vi "Continue Read.vi"(8 "error in":errorcluster, 11 "Com in":refnum<visa-resource-name>) -> (0 "error out":errorcluster, 2 "Data":i64[](array[numeric]), 3 "Com out":refnum<visa-resource-name>)   [LabVIEW 2020]
panel:
  out "read buffer":string
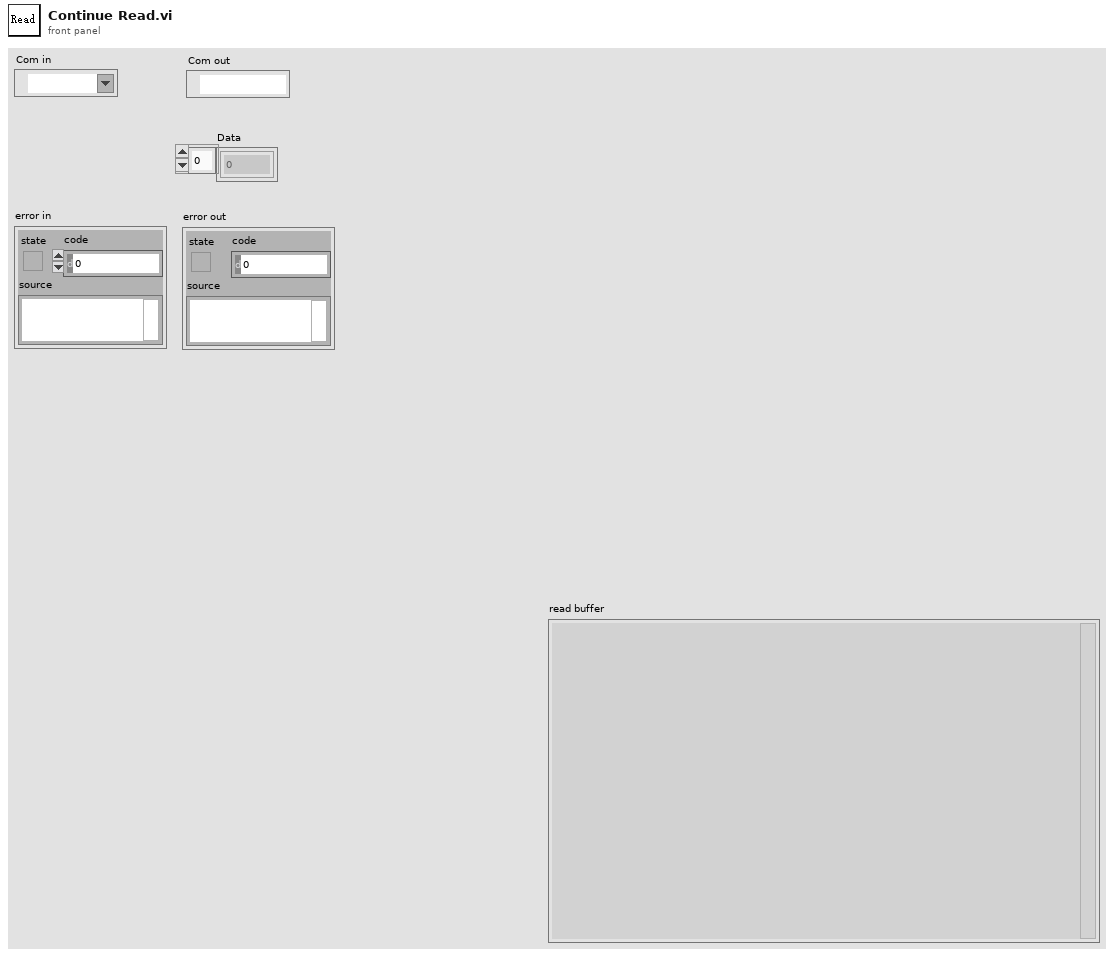
[diagram p1: front panel]
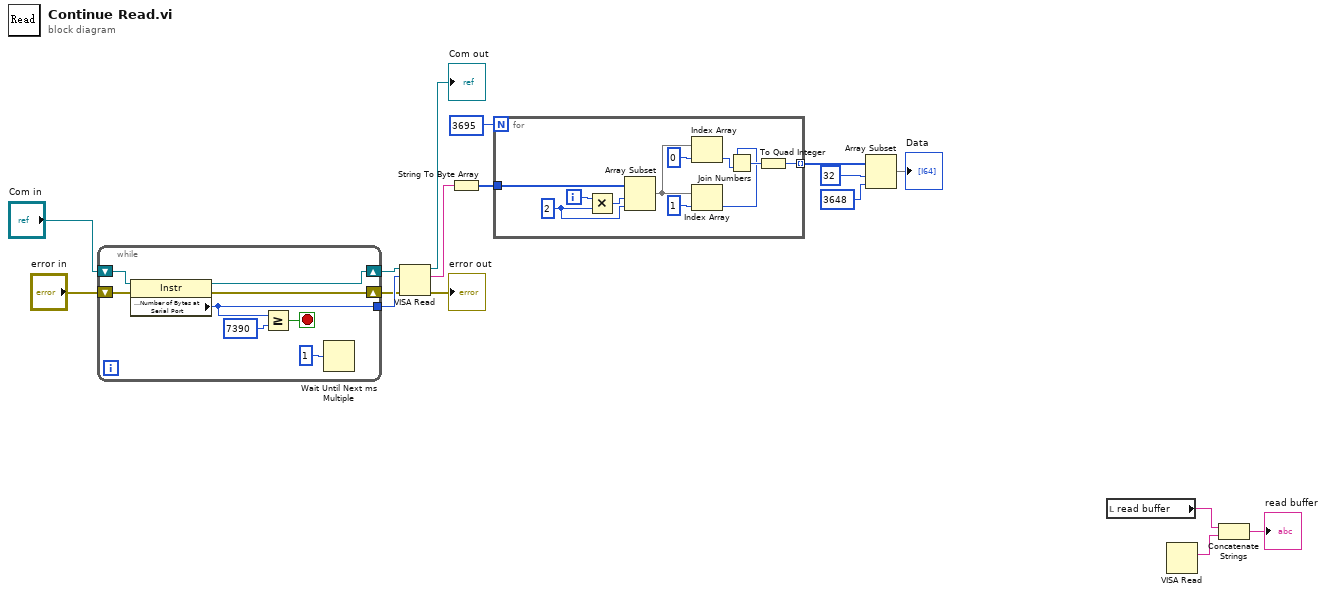
[diagram p0: block diagram]
diagram:
  n1 = while {
    tunnel: [w23] -> w18
    shift-right: [w26] -> w17
    shift-left: "error in" -> [w25]
    shift-right: [w27] -> w19
    shift-left: "Com in" -> [w24]
    stop <- w22 stop-if-true
    n2 = property class="Instr"(reference=w24, error in=w25) -> (reference out=w27:refnum<visa-resource-name>, error out=w26:errorcluster, "Serial Settings:Number of Bytes at Serial Port"=w23:u32)
    n3 = Greater Or Equal?(x=w23, y=u32 7390) -> (x >= y?=w22:bool)
    n4 = Wait Until Next ms Multiple(millisecond multiple=u32 1 ("毫秒倍数")) -> ()  [unwired: 1 out]
  }
  n5 = VISA Read(VISA resource name=w19, byte count=w18, error in (no error)=w17) -> (VISA resource name out=→"Com out":refnum<visa-resource-name>, read buffer=w16:string, error out=→"error out":errorcluster)  [unwired: 1 out]
  n6 = String To Byte Array(string=w16) -> (unsigned byte array=w15:u8[])
  n7 = for {
    N: 3695 -> [_]
    tunnel: w15 -> [w38]
    tunnel: [w30] -> w13 mode=indexing
    i -> [w36]
    w35 = 2 ("长度")
    n8 = Multiply(x=w36, y=w35) -> (x*y=w37:i32)
    n9 = Array Subset(array=w38, index=w37, length=w35) -> (w34:u8[])
    n10 = Index Array(array=w34, index=0 ("索引")) -> (element=w29:u8)
    n11 = Index Array(array=w34, index=1 ("索引")) -> (element=w28:u8)
    n12 = Join Numbers(hi=w28, lo=w29) -> ((hi.lo)=w31:u16)
    n13 = To Quad Integer(1:w31) -> (0:w30:i64)
  }
  n14 = Array Subset(array=w13, index=32 ("索引"), length=3648 ("长度")) -> (→"Data":i64[])
  n15 = local read "read buffer"() -> (w1:string)
  n16 = VISA Read() -> (VISA resource name=w5:refnum<visa-resource-name>, byte count=w4:u32, read buffer=w2:string)  [unwired: 1 in, 3 out]
  n17 = Concatenate Strings(w1, w2) -> (→"read buffer":string)
